vi "xmlData.vi"(10 "Array":string[](array[string]), 11 "Numeric":i32) -> ()   [LabVIEW 2018]
uses:
  Global Variables.vi
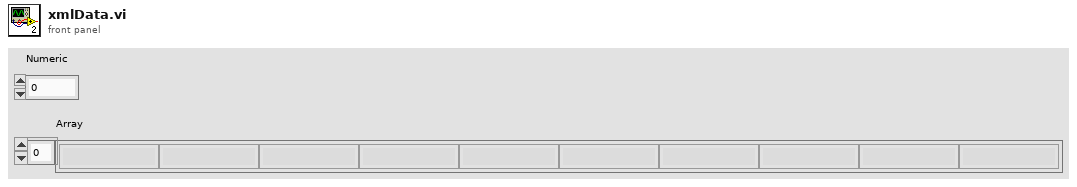
[diagram p1: front panel]
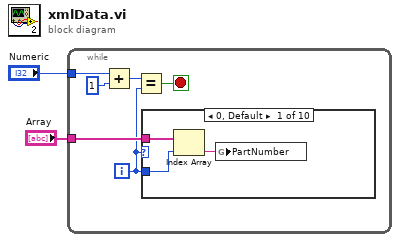
[diagram p0: block diagram]
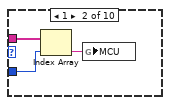
[diagram p2: hidden frame]
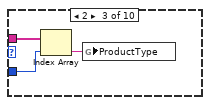
[diagram p3: hidden frame]
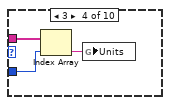
[diagram p4: hidden frame]
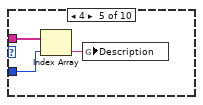
[diagram p5: hidden frame]
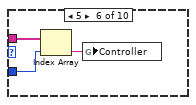
[diagram p6: hidden frame]
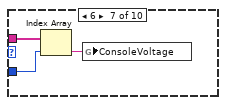
[diagram p7: hidden frame]
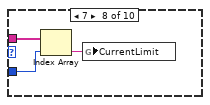
[diagram p8: hidden frame]
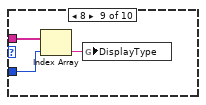
[diagram p9: hidden frame]
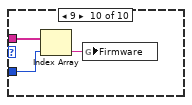
[diagram p10: hidden frame]
diagram:
  n1 = while {
    tunnel: "Array" -> [w7]
    tunnel: "Numeric" -> [w5]
    i -> [w6]
    stop <- w8 stop-if-true
    n2 = Add(x=w5, y=1) -> (x+y=w4:i32)
    n3 = Equal?(x=w4, y=w6) -> (x = y?=w8:bool)
    n4 = case shown="0, Default" w6 {
      tunnel: w7 -> [w11 w14 w17 w20 w23 w26 w29 w32 w35 w38]
      tunnel: w6 -> [w10 w13 w16 w19 w22 w25 w28 w31 w34 w37]
      frame 0, Default {
        n5 = Index Array(array=w11, index=w10) -> (element=w9:string)
        n6 = global write "Global Variables.vi" "PartNumber"(w9) -> ()
      }
      frame 1 {
        n7 = Index Array(array=w14, index=w13) -> (element=w12:string)
        n8 = global write "Global Variables.vi" "MCU"(w12) -> ()
      }
      frame 2 {
        n9 = Index Array(array=w17, index=w16) -> (element=w15:string)
        n10 = global write "Global Variables.vi" "ProductType"(w15) -> ()
      }
      frame 3 {
        n11 = Index Array(array=w20, index=w19) -> (element=w18:string)
        n12 = global write "Global Variables.vi" "Units"(w18) -> ()
      }
      frame 4 {
        n13 = Index Array(array=w23, index=w22) -> (element=w21:string)
        n14 = global write "Global Variables.vi" "Description"(w21) -> ()
      }
      frame 5 {
        n15 = Index Array(array=w26, index=w25) -> (element=w24:string)
        n16 = global write "Global Variables.vi" "Controller"(w24) -> ()
      }
      frame 6 {
        n17 = Index Array(array=w29, index=w28) -> (element=w27:string)
        n18 = global write "Global Variables.vi" "ConsoleVoltage"(w27) -> ()
      }
      frame 7 {
        n19 = Index Array(array=w32, index=w31) -> (element=w30:string)
        n20 = global write "Global Variables.vi" "CurrentLimit"(w30) -> ()
      }
      frame 8 {
        n21 = Index Array(array=w35, index=w34) -> (element=w33:string)
        n22 = global write "Global Variables.vi" "DisplayType"(w33) -> ()
      }
      frame 9 {
        n23 = Index Array(array=w38, index=w37) -> (element=w36:string)
        n24 = global write "Global Variables.vi" "Firmware"(w36) -> ()
      }
    }
  }
